vi "GetClassPrivateDataClusterRef.vi"(8 "error in (no error)":errorcluster, 11 "LVClassLibrary Ref":refnum<vi>) -> (0 "error out":errorcluster, 1 "Class private data cluster refnum":refnum<vi>, 2 "Class private data vi refnum":refnum<vi>, 3 "LVClassLibrary Ref":refnum<vi>)   [LabVIEW 2019, in "BlueUtilityScripts.lvlib"]
uses:
  BlueUtilityScripts.lvlib
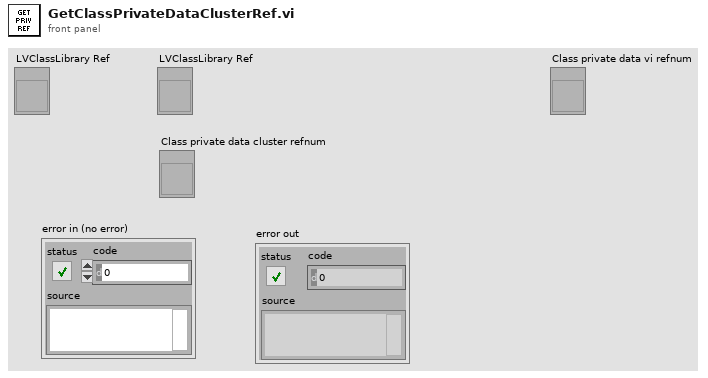
[diagram p1: front panel]
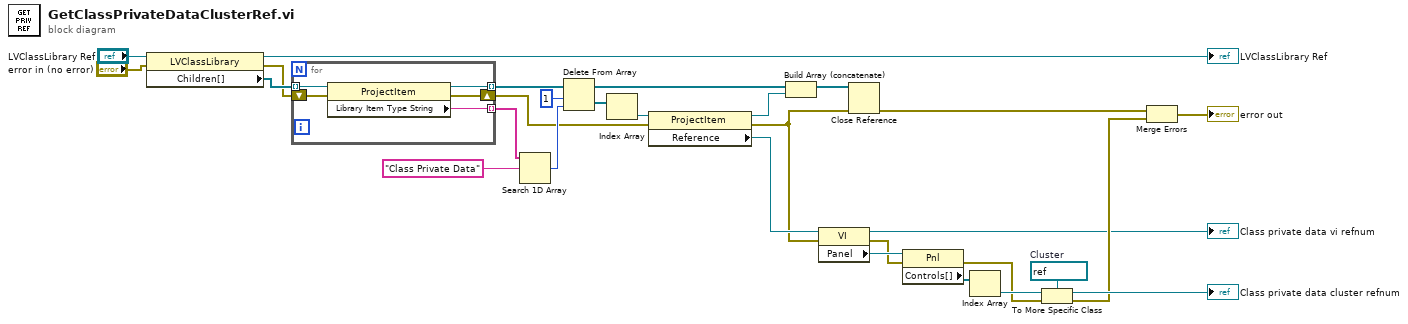
[diagram p0: block diagram]
diagram:
  w12 = refnum<vi> refnum  # Cluster
  n1 = property class="LVClassLibrary"(reference="LVClassLibrary Ref", error in="error in (no error)") -> (reference out=→"LVClassLibrary Ref":refnum<vi>, error out=w21:errorcluster, "Children[]"=w29:refnum<vi>[])
  n2 = for {
    tunnel: w29 -> [w34] mode=indexing
    tunnel: [w33] -> w28 mode=indexing
    tunnel: [w32] -> w26 mode=indexing
    shift-right: [w30] -> w20
    shift-left: w21 -> [w31]
    n3 = property class="ProjectItem"(reference=w34, error in=w31) -> (reference out=w32:refnum<vi>, error out=w30:errorcluster, "Library Item Type String"=w33:string)
  }
  n4 = Search 1D Array(1D array=w28, element="Class Private Data" ("Library Item Type String")) -> (index of element=w24:i32)  [unwired: 1 out]
  n5 = Delete From Array(array=w26, length=1, index=w24) -> (deleted portion=w23:refnum<vi>[], array with subset deleted=w18:refnum<vi>[])
  n6 = Index Array(array=w23) -> (element=w22:refnum<vi>)  [unwired: 1 in]
  n7 = property class="ProjectItem"(reference=w22, error in=w20) -> (reference out=w19:refnum<vi>, error out=w11:errorcluster, "Reference"=w16:refnum<vi>)
  n8 = Build Array (concatenate)(w18, w19) -> (w17:refnum<vi>[])
  n9 = property class="VI"(reference=w16, error in=w11) -> (reference out=→"Class private data vi refnum":refnum<vi>, error out=w10:errorcluster, "Panel"=w15:refnum<vi>)
  n10 = Close Reference(reference=w17, error in (no error)=w11) -> (error out=w4:errorcluster)
  n11 = property class="Pnl"(reference=w15, error in=w10) -> (error out=w9:errorcluster, "Controls[]"=w14:refnum<vi>[])  [unwired: 1 out]
  n12 = Index Array(array=w14) -> (element=w13:refnum<vi>)  [unwired: 1 in]
  n13 = To More Specific Class(target class=w12, reference=w13, error in=w9) -> (specific class reference=→"Class private data cluster refnum":refnum<vi>, error out=w3:errorcluster)
  n14 = Merge Errors(w4, w3) -> (→"error out":errorcluster)
